vi "Add Language.vi"(8 "error in (no error)":errorcluster, 11 "Controller in":refnum<class "Controller.lvclass">) -> (0 "error out":errorcluster, 3 "Controller out":refnum<class "Controller.lvclass">)   [LabVIEW 2013, in "SET Project Editor.lvlib" / "Controller.lvclass"]
uses:
  Controller.lvclass
  Controller.lvclass/Controller.ctl
  SET Project Data/Project Data Class/Project Data.lvclass
  <vilib>/ActorFramework/Message Enqueuer/Message Enqueuer.lvclass/Message Enqueuer.ctl
  <vilib>/ActorFramework/Message Enqueuer/Enqueue.vi
  <vilib>/ActorFramework/Message Priority Queue/Priority Enqueue.vi
  SET Project Data/Resource Data Class/Resource Data.lvclass
  UI View Messages/UI Refresh Data Msg/UI Refresh Data Msg.lvclass
  SET Project Editor.lvlib
  SET Project Data/SET Project Data.lvlib
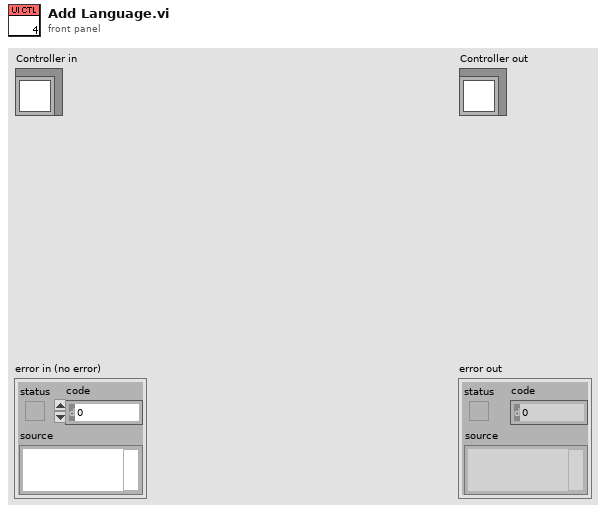
[diagram p1: front panel]
types:
  T1 = typedef "SET Project Data.lvlib/ProjFile_Language Entry.ctl" = cluster{"Tag":string, "Name":string, "Code Page":u16}
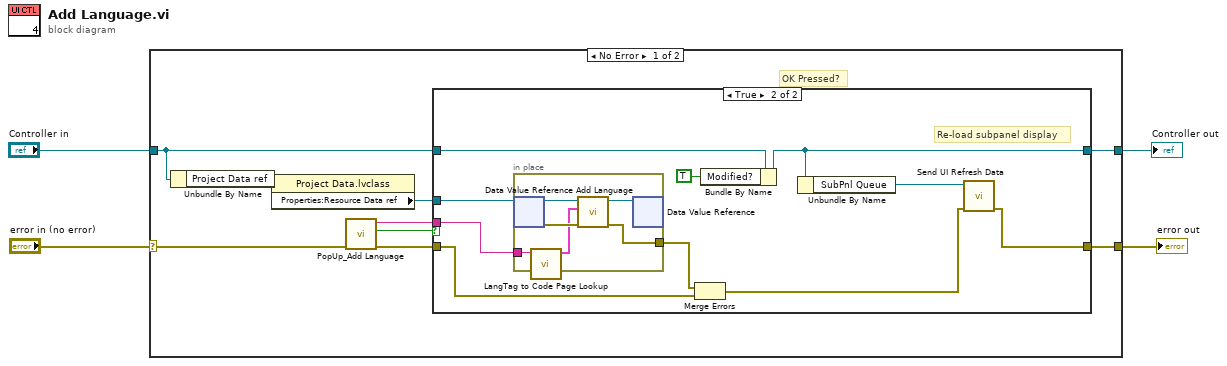
[diagram p0: block diagram]
diagram:
  n1 = case shown="No Error" "error in (no error)" {
    selector: "error in (no error)" -> [w11 w33]
    tunnel: [w12 w33] -> w2
    tunnel: [w13 w32] -> w1
    tunnel: "Controller in" -> [w7 w32]
    frame No Error {
      # "OK Pressed?"
      n2 = Unbundle By Name(w7) -> ("Project Data ref"=w6:refnum<data-value>)
      n3 = property class="Project Data.lvclass"(reference=w6) -> ("Properties:Resource Data ref"=w5:refnum<data-value>)  [unwired: 1 in, 2 out]
      n4 = call "PopUp_Add Language.vi"("error in (no error)"=w11) -> ("error out"=w10:errorcluster, "OK Pressed?"=w8:bool, "NewLang Name"=w9:string)  [unwired: 8 in]
      n5 = case shown="True" w8 {
        tunnel: w7 -> [w15 w21]
        tunnel: [w15 w19] -> w13
        tunnel: [w14 w16] -> w12
        tunnel: w10 -> [w14 w24]
        tunnel: w9 -> [_ w22]
        tunnel: w5 -> [_ w23]
        frame False {
        }
        frame True {
          # "Re-load subpanel display"
          n6 = in-place {
            in-place-border: w22 -> [w27]
            in-place-border: [w28] -> w25
            n7 = in-place-dvr #1(w23) -> (w31:refnum<class "Resource Data.lvclass">, w29:errorcluster)
            n8 = call "LangTag to Code Page Lookup.vi"("Tag"=w27) -> ("Language"=w26:T1)  [unwired: 9 in, 1 out]
            n9 = call "Add Language.vi"("error in (no error)"=w29, "Language"=w26, "LangFile in"=w31) -> ("error out"=w28:errorcluster, "LangFile out"=w30:refnum<class "Resource Data.lvclass">)  [unwired: 7 in]
            n10 = in-place-dvr #1(w30) -> ()  [unwired: 2 out]
          }
          n11 = Merge Errors(w25, w24) -> (w17:errorcluster)
          n12 = Bundle By Name(cluster=w21, "Modified?"=TRUE) -> (w19:refnum<class "Controller.lvclass">)
          n13 = Unbundle By Name(w19) -> ("SubPnl Queue"=w18:refnum<class "Message Enqueuer.lvclass">)
          n14 = call "Send UI Refresh Data.vi"("error in (no error)"=w17, "Message Enqueuer"=w18) -> ("error out"=w16:errorcluster)  [unwired: 8 in, 1 out]
        }
      }
    }
    frame Error {
    }
  }
  "error out" <- w2
  "Controller out" <- w1
